vi "Get XAPI Path.vi"() -> (0 "XAPI Library Path":path)   [LabVIEW 2018, in "Fujifilm X Series GFX System Digital Camera.lvlib"]
uses:
  <instrlib>/Fujifilm X Series GFX System Digital Camera/Fujifilm X Series GFX System Digital Camera.lvlib
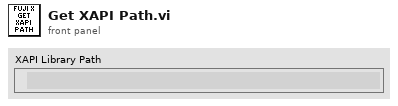
[diagram p1: front panel]
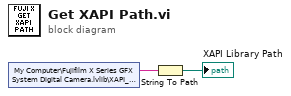
[diagram p0: block diagram]
diagram:
  n1 = shared-variable "My Computer\\Fujifilm X Series GFX System Digital Camera.lvlib\\XAPI_SDK_PATH"() -> (w2:string)  [unwired: 1 in, 1 out]
  n2 = String To Path(string=w2) -> (path=→"XAPI Library Path":path)
